vi "Delete Elements from Array__ogtk.vi"   [LabVIEW 2012]
doc: "This polymorphic VI deletes elements from a 1D or 2D <B>array</B> at the corresponding <B>indices</B>, returning <B>array w/ subset deleted</B> and <B>deleted elements</B>. For 2D arrays, wire the <B>delete (rows or columns)</B> input to specify whether to delete rows or columns."
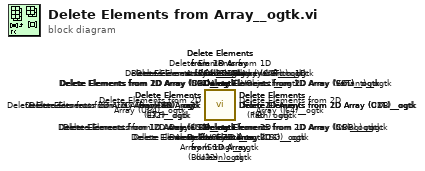
[diagram p0: block diagram]
diagram:
  n1 = call <userlib>:"Delete Elements from 2D Array (LVObject)__ogtk.vi"() -> ()  [unwired: 10 in, 2 out]
  n2 = call <userlib>:"Delete Elements from 1D Array (LVObject)__ogtk.vi"() -> ()  [unwired: 10 in, 2 out]
  n3 = call <userlib>:"Delete Elements from 2D Array (U64)__ogtk.vi"() -> ()  [unwired: 10 in, 2 out]
  n4 = call <userlib>:"Delete Elements from 2D Array (I64)__ogtk.vi"() -> ()  [unwired: 10 in, 2 out]
  n5 = call <userlib>:"Delete Elements from 1D Array (U64)__ogtk.vi"() -> ()  [unwired: 10 in, 2 out]
  n6 = call <userlib>:"Delete Elements from 1D Array (I64)__ogtk.vi"() -> ()  [unwired: 10 in, 2 out]
  n7 = call <userlib>:"Delete Elements from 1D Array (Boolean)__ogtk.vi"() -> ()  [unwired: 10 in, 2 out]
  n8 = call <userlib>:"Delete Elements from 1D Array (CDB)__ogtk.vi"() -> ()  [unwired: 10 in, 2 out]
  n9 = call <userlib>:"Delete Elements from 1D Array (CSG)__ogtk.vi"() -> ()  [unwired: 10 in, 2 out]
  n10 = call <userlib>:"Delete Elements from 1D Array (DBL)__ogtk.vi"() -> ()  [unwired: 10 in, 2 out]
  n11 = call <userlib>:"Delete Elements from 1D Array (CXT)__ogtk.vi"() -> ()  [unwired: 10 in, 2 out]
  n12 = call <userlib>:"Delete Elements from 1D Array (EXT)__ogtk.vi"() -> ()  [unwired: 10 in, 2 out]
  n13 = call <userlib>:"Delete Elements from 1D Array (I8)__ogtk.vi"() -> ()  [unwired: 10 in, 2 out]
  n14 = call <userlib>:"Delete Elements from 1D Array (I16)__ogtk.vi"() -> ()  [unwired: 10 in, 2 out]
  n15 = call <userlib>:"Delete Elements from 1D Array (I32)__ogtk.vi"() -> ()  [unwired: 10 in, 2 out]
  n16 = call <userlib>:"Delete Elements from 1D Array (Path)__ogtk.vi"() -> ()  [unwired: 10 in, 2 out]
  n17 = call <userlib>:"Delete Elements from 1D Array (SGL)__ogtk.vi"() -> ()  [unwired: 10 in, 2 out]
  n18 = call <userlib>:"Delete Elements from 1D Array (String)__ogtk.vi"() -> ()  [unwired: 10 in, 2 out]
  n19 = call <userlib>:"Delete Elements from 1D Array (U8)__ogtk.vi"() -> ()  [unwired: 10 in, 2 out]
  n20 = call <userlib>:"Delete Elements from 1D Array (U16)__ogtk.vi"() -> ()  [unwired: 10 in, 2 out]
  n21 = call <userlib>:"Delete Elements from 1D Array (U32)__ogtk.vi"() -> ()  [unwired: 10 in, 2 out]
  n22 = call <userlib>:"Delete Elements from 1D Array (Variant)__ogtk.vi"() -> ()  [unwired: 10 in, 2 out]
  n23 = call <userlib>:"Delete Elements from 2D Array (Boolean)__ogtk.vi"() -> ()  [unwired: 10 in, 2 out]
  n24 = call <userlib>:"Delete Elements from 2D Array (CDB)__ogtk.vi"() -> ()  [unwired: 10 in, 2 out]
  n25 = call <userlib>:"Delete Elements from 2D Array (CSG)__ogtk.vi"() -> ()  [unwired: 10 in, 2 out]
  n26 = call <userlib>:"Delete Elements from 2D Array (CXT)__ogtk.vi"() -> ()  [unwired: 10 in, 2 out]
  n27 = call <userlib>:"Delete Elements from 2D Array (DBL)__ogtk.vi"() -> ()  [unwired: 10 in, 2 out]
  n28 = call <userlib>:"Delete Elements from 2D Array (EXT)__ogtk.vi"() -> ()  [unwired: 10 in, 2 out]
  n29 = call <userlib>:"Delete Elements from 2D Array (I8)__ogtk.vi"() -> ()  [unwired: 10 in, 2 out]
  n30 = call <userlib>:"Delete Elements from 2D Array (I16)__ogtk.vi"() -> ()  [unwired: 10 in, 2 out]
  n31 = call <userlib>:"Delete Elements from 2D Array (I32)__ogtk.vi"() -> ()  [unwired: 10 in, 2 out]
  n32 = call <userlib>:"Delete Elements from 2D Array (Path)__ogtk.vi"() -> ()  [unwired: 10 in, 2 out]
  n33 = call <userlib>:"Delete Elements from 2D Array (SGL)__ogtk.vi"() -> ()  [unwired: 10 in, 2 out]
  n34 = call <userlib>:"Delete Elements from 2D Array (String)__ogtk.vi"() -> ()  [unwired: 10 in, 2 out]
  n35 = call <userlib>:"Delete Elements from 2D Array (U8)__ogtk.vi"() -> ()  [unwired: 10 in, 2 out]
  n36 = call <userlib>:"Delete Elements from 2D Array (U16)__ogtk.vi"() -> ()  [unwired: 10 in, 2 out]
  n37 = call <userlib>:"Delete Elements from 2D Array (U32)__ogtk.vi"() -> ()  [unwired: 10 in, 2 out]
  n38 = call <userlib>:"Delete Elements from 2D Array (Variant)__ogtk.vi"() -> ()  [unwired: 10 in, 2 out]
